vi "Restore Format Property.vi"(4 "Control Ref Cluster":T1, 6 "Update?":bool=TRUE, 7 "Polor?":bool, 8 "error in (no error)":errorcluster, 11 "2D Plot.lvclass in":refnum<class "2D Plot.lvclass">) -> (0 "error out":errorcluster, 3 "2D Plot.lvclass out":refnum<class "2D Plot.lvclass">)   [LabVIEW 2017, in "2D Plot.lvclass"]
uses:
  <vilib>/Math Plots/2D Math Plots/2D Plot/2D Plot/2D Plot.lvclass
  <vilib>/Math Plots/2D Math Plots/2D Plot/Action String/2DMathPlot Ctrl Act Cluster.ctl
  <vilib>/Math Plots/2D Math Plots/2D Plot/Action String/2DMathPlot State Class.ctl
  <vilib>/Math Plots/2D Math Plots/2D Plot/2D Plot/2D Plot.lvclass/2D Plot.ctl
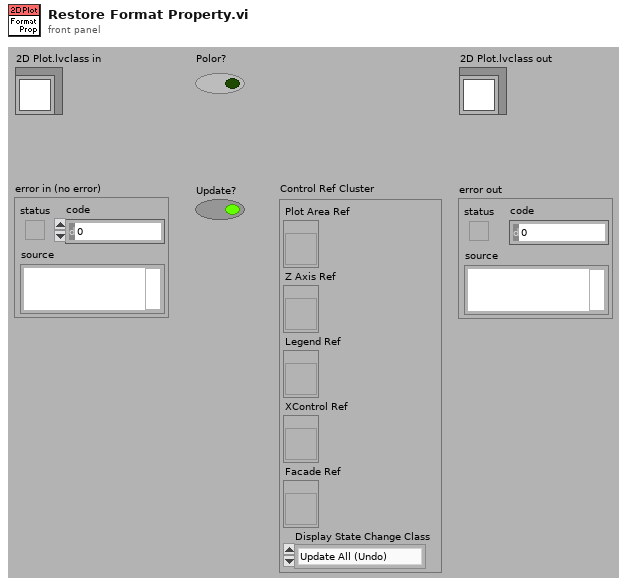
[diagram p1: front panel]
types:
  T1 = typedef "2DMathPlot Ctrl Act Cluster.ctl" = cluster{"Plot Area Ref":refnum<vi>, "Z Axis Ref":refnum<vi>, "Legend Ref":refnum<vi>, "XControl Ref":refnum<vi>, "Facade Ref":refnum<vi>, "Display State Change Class":T2}
  T2 = typedef "2DMathPlot State Class.ctl" = enum16{"Update All (Undo)", "Update General", "Update Appearance", "Update Format", "Update Scale", "Update Marker", "Update Cursor", "None"}
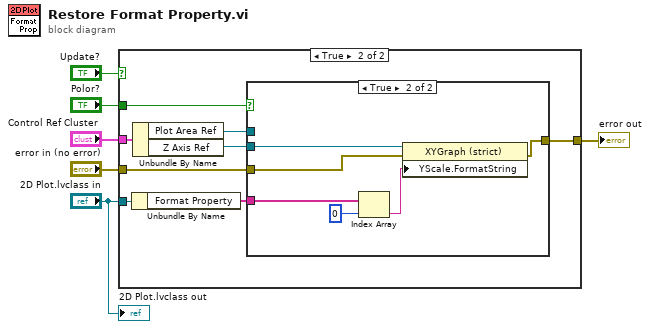
[diagram p0: block diagram]
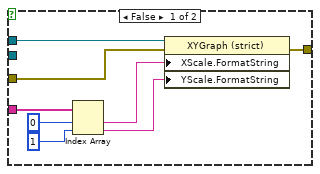
[diagram p3: hidden frame]
diagram:
  n1 = case shown="True" "Update?" {
    tunnel: "2D Plot.lvclass in" -> [_ w15]
    tunnel: "Control Ref Cluster" -> [_ w13]
    tunnel: "Polor?" -> [_ w10]
    tunnel: "error in (no error)" -> [w7 w9]
    tunnel: [w7 w8] -> w2
    frame False {
    }
    frame True {
      n2 = Unbundle By Name(w15) -> ("Format Property"=w14:string[])
      n3 = Unbundle By Name(w13) -> ("Plot Area Ref"=w12:refnum<vi>, "Z Axis Ref"=w11:refnum<vi>)
      n4 = case shown="True" w10 {
        tunnel: [w20 w28] -> w8
        tunnel: w14 -> [w23 w25]
        tunnel: w12 -> [w22 _]
        tunnel: w11 -> [_ w27]
        tunnel: w9 -> [w21 w26]
        frame False {
          n5 = Index Array(array=w23, index #1=0 ("index"), index #2=1 ("index")) -> (element #1=w19:string, element #2=w18:string)
          n6 = property class="XYGraph (strict)"(reference=w22, error in=w21, "XScale.FormatString"=w19, "YScale.FormatString"=w18) -> (error out=w20:errorcluster)  [unwired: 1 out]
        }
        frame True {
          n7 = Index Array(array=w25, index=0) -> (element=w29:string)
          n8 = property class="XYGraph (strict)"(reference=w27, error in=w26, "YScale.FormatString"=w29) -> (error out=w28:errorcluster)  [unwired: 1 out]
        }
      }
    }
  }
  "error out" <- w2
  "2D Plot.lvclass out" <- "2D Plot.lvclass in"
